vi "Data_Preparation.vi"(0 "File Path":path=path "E:/Documents/LabVIEW/EEG/Filtered_Data/s01_ex01_s01.csv") -> (1 "Header":string[](array[string]), 2 "Datas":dbl[][](array[numeric]))   [LabVIEW 2023]
uses:
  <vilib>/Utility/file.llb/Read Delimited Spreadsheet (DBL).vi
  <vilib>/Utility/file.llb/Read Delimited Spreadsheet (string).vi
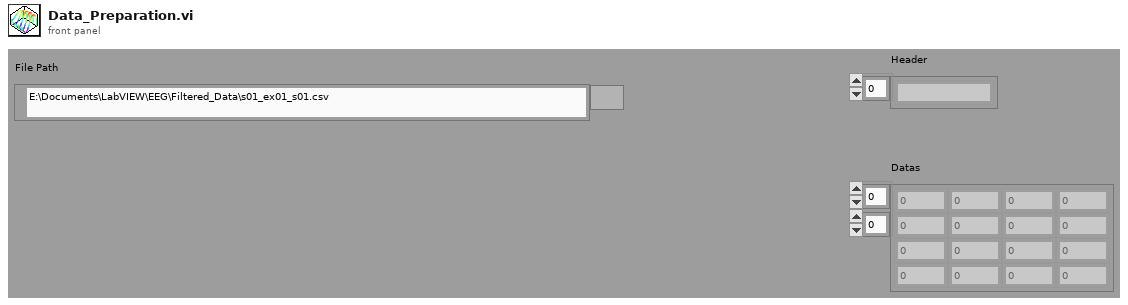
[diagram p1: front panel]
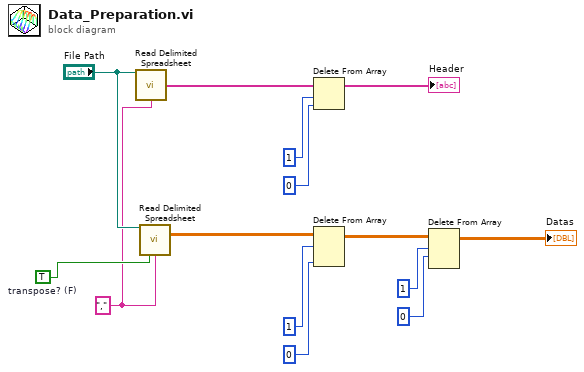
[diagram p0: block diagram]
diagram:
  w12 = TRUE  # transpose? (F)
  w1 = "," ("delimiter (\\t)")
  n1 = call-poly <vilib>:"Read Delimited Spreadsheet.vi"("file path (dialog if empty)"="File Path", "delimiter (\\t)"=w1) -> ("first row"=w8:string[])  [unwired: 8 in, 5 out]
  n2 = call-poly <vilib>:"Read Delimited Spreadsheet.vi"("file path (dialog if empty)"="File Path", "transpose? (F)"=w12, "delimiter (\\t)"=w1) -> ("all rows"=w2:dbl[][])  [unwired: 7 in, 5 out]
  n3 = Delete From Array "Delete From Array"(array=w8, length=1, index=0) -> (array with subset deleted=→"Header":string[])  [unwired: 1 out]
  n4 = Delete From Array "Delete From Array"(array=w2, length=1, index (col)=0) -> (array with subset deleted=w5:dbl[][])  [unwired: 1 in, 1 out]
  n5 = Delete From Array "Delete From Array"(array=w5, length=1, index (row)=0) -> (array with subset deleted=→"Datas":dbl[][])  [unwired: 1 in, 1 out]
